vi "simx Pause Communication.vi"(8 "error in (no error)":errorcluster, 10 "pause":u8, 11 "clientID":i32) -> (0 "error out":errorcluster, 3 "function return":i32)   [LabVIEW 2019, in "PXL_V-REP.lvlib"]
doc: "EXTAPI_DLLEXPORT simxInt simxPauseCommunication(simxInt clientID,simxUChar pause);"
uses:
  PXL_V-REP.lvlib
  <userlib>/V-REP/remoteApi.dll
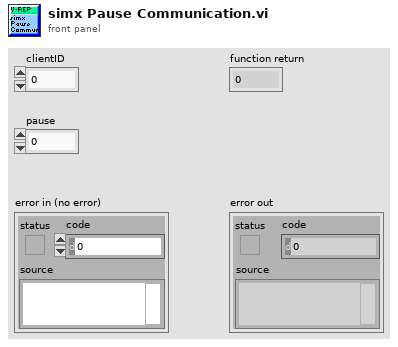
[diagram p1: front panel]
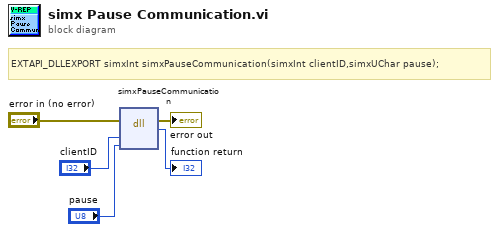
[diagram p0: block diagram]
diagram:
  # "EXTAPI_DLLEXPORT simxInt simxPauseCommunication(simxInt clientID,simxUChar pause);"
  n1 = dll-call lib="C:/Program Files (x86)/National Instruments/LabVIEW 2019/user.lib/V-REP/remoteApi.*" fn="simxPauseCommunication"(error in="error in (no error)", "clientID"="clientID", "pause"="pause") -> (error out=→"error out":errorcluster, →"function return":i32)  [unwired: 4 in, 1 out]
